vi "dfd_Convert Coef Quantizer to String.vi"(7 "indent order":i32, 10 "quantizer name":string="Quantizer ", 11 "quantization settings":T1={"source"=0, "wl"=16, "iwl"=1, "overflow mode"=enum."Saturation", "rounding mode"=enum."Nearest", "signed?"=TRUE} {"source" items=["Coef a/k"=0, "Coef b/v"=7, "Input"=1, "Output"=2, "Multiplicand"=3, "Product"=4, "Sum"=5, "Delay"=6, "Gain"=8]}) -> (3 "xml string out":string)   [LabVIEW 2017, in "NI_DigFilter_Process.lvlib"]
uses:
  <vilib>/addons/Digital Filter Design/NI_DigFilter_Process.lvlib
  <vilib>/addons/Digital Filter Design/_Objects.llb/dfd_Internal Quantization Settings.ctl
  <vilib>/addons/Digital Filter Design/_Objects.llb/dfd_Internal Quantization Srcs.ctl
  <vilib>/addons/Digital Filter Design/NI_DigFilterLicensed.lvlib
panel:
  out "q_mode":enum16{"Nearest", "Truncation"}(ring)
  out "o_mode":enum16{"Saturation", "Wrap"}(ring)
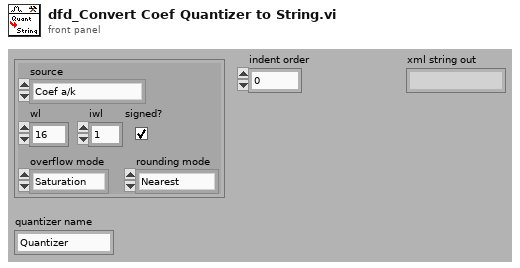
[diagram p1: front panel]
types:
  T1 = typedef "NI_DigFilterLicensed.lvlib/dfd_Internal Quantization Settings.ctl" = cluster{"source":T2, "wl":i16, "iwl":i16, "overflow mode":enum16{"Saturation", "Wrap"}, "rounding mode":enum16{"Nearest", "Truncation"}, "signed?":bool}
  T2 = typedef "NI_DigFilterLicensed.lvlib/dfd_Internal Quantization Srcs.ctl" = u16
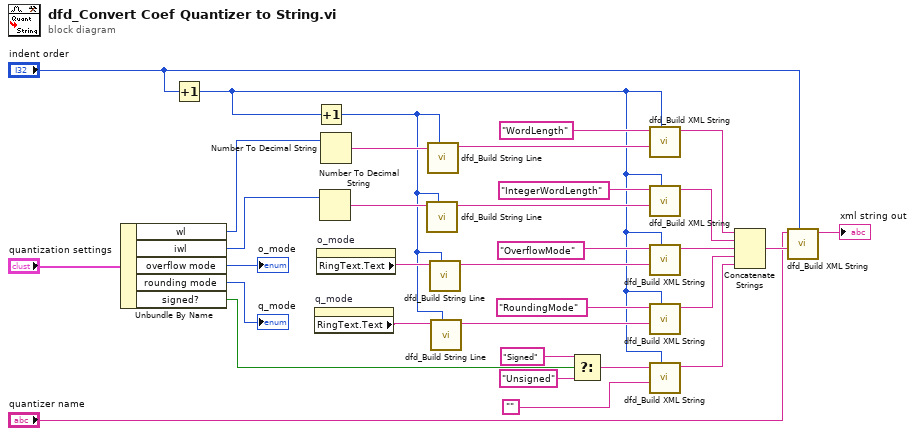
[diagram p0: block diagram]
diagram:
  n1 = Unbundle By Name("quantization settings") -> ("wl"=w1:i16, "iwl"=w32:i16, "overflow mode"=→"o_mode":enum16{"Saturation", "Wrap"}, "rounding mode"=→"q_mode":enum16{"Nearest", "Truncation"}, "signed?"=w26:bool)
  n2 = Increment(x="indent order") -> (x+1=w4:i32)
  n3 = property on="q_mode" class="Enum (strict)"() -> ("RingText.Text"=w10:string)  [unwired: 2 in, 2 out]
  n4 = Increment(x=w4) -> (x+1=w8:i32)
  n5 = property on="o_mode" class="Enum (strict)"() -> ("RingText.Text"=w12:string)  [unwired: 2 in, 2 out]
  n6 = Number To Decimal String(number=w32) -> (decimal integer string=w14:string)  [unwired: 1 out]
  n7 = Number To Decimal String(number=w1) -> (decimal integer string=w16:string)  [unwired: 1 out]
  n8 = call <vilib>:"dfd_Build String Line.vi"("indent order"=w8, "string"=w14) -> ("string line"=w13:string)  [unwired: 9 out]
  n9 = call <vilib>:"dfd_Build String Line.vi"("indent order"=w8, "string"=w16) -> ("string line"=w15:string)  [unwired: 9 out]
  n10 = call <vilib>:"dfd_Build String Line.vi"("indent order"=w8, "string"=w12) -> ("string line"=w11:string)  [unwired: 9 out]
  n11 = call <vilib>:"dfd_Build String Line.vi"("indent order"=w8, "string"=w10) -> ("string line"=w9:string)  [unwired: 9 out]
  n12 = Select(t="Signed", s=w26, f="Unsigned") -> (s? t:f=w24:string)
  n13 = call <vilib>:"dfd_Build XML String.vi"("indent order"=w4, "string in"=w15, "element name"="WordLength") -> ("xml string out"=w21:string)  [unwired: 1 in, 7 out]
  n14 = call <vilib>:"dfd_Build XML String.vi"("indent order"=w4, "string in"=w13, "element name"="IntegerWordLength") -> ("xml string out"=w20:string)  [unwired: 1 in, 7 out]
  n15 = call <vilib>:"dfd_Build XML String.vi"("indent order"=w4, "string in"=w11, "element name"="OverflowMode") -> ("xml string out"=w19:string)  [unwired: 1 in, 7 out]
  n16 = call <vilib>:"dfd_Build XML String.vi"("indent order"=w4, "string in"=w9, "element name"="RoundingMode") -> ("xml string out"=w18:string)  [unwired: 1 in, 7 out]
  n17 = call <vilib>:"dfd_Build XML String.vi"("indent order"=w4, "string in"="", "element name"=w24) -> ("xml string out"=w17:string)  [unwired: 1 in, 7 out]
  n18 = Concatenate Strings(w21, w20, w19, w18, w17) -> (w6:string)
  n19 = call <vilib>:"dfd_Build XML String.vi"("indent order"="indent order", "string in"=w6, "element name"="quantizer name") -> ("xml string out"=→"xml string out":string)  [unwired: 1 in, 7 out]
